vi "Check Code.vi"(11 "Code":string[][](array[string])) -> (3 "Code Good":bool)   [LabVIEW 2011]
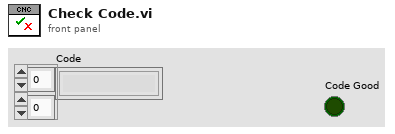
[diagram p1: front panel]
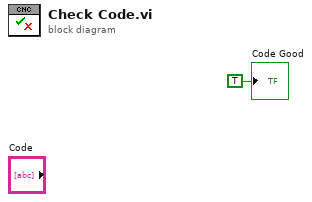
[diagram p0: block diagram]
diagram:
  "Code Good" <- TRUE ("Code Good")
